vi "Get CDs NodeIDs by GUID.vi"(8 "error in (no error)":errorcluster, 10 "Custom Device GUID":string, 11 "Target ref in":refnum<k24>) -> (0 "error out":errorcluster, 2 "NodeIDs":u64[](array[numeric]), 3 "Target ref out":refnum<k24>)   [LabVIEW 2019, in "TLCD Test.lvclass"]
uses:
  TLCD Test.lvclass
  NationalInstruments.VeriStand.SystemDefinitionAPI
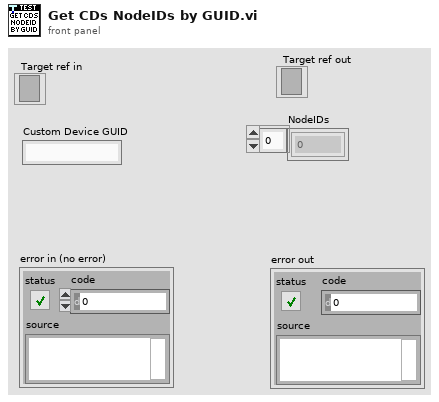
[diagram p1: front panel]
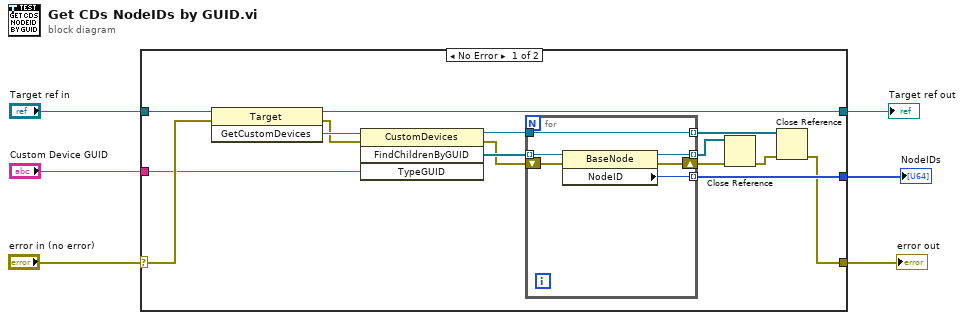
[diagram p0: block diagram]
diagram:
  n1 = case shown="No Error" "error in (no error)" {
    selector: "error in (no error)" -> [w20 w28]
    tunnel: "Target ref in" -> [w21 w29]
    tunnel: [w16 w29] -> w5
    tunnel: [w7 w28] -> w4
    tunnel: "Custom Device GUID" -> [w18 _]
    tunnel: [w13 _] -> w1
    frame No Error {
      n2 = invoke class="Target" method="GetCustomDevices"(reference=w21, error in=w20) -> (reference out=w16:refnum<k24>, error out=w17:errorcluster, "GetCustomDevices"=w19:refnum<k24>)  [unwired: 1 in]
      n3 = invoke class="CustomDevices" method="FindChildrenByGUID"(reference=w19, error in=w17, "TypeGUID"=w18) -> (reference out=w10:refnum<k24>, error out=w14:errorcluster, "FindChildrenByGUID"=w15:refnum<k24>[])  [unwired: 1 in, 1 out]
      n4 = for {
        tunnel: w15 -> [w27] mode=indexing
        tunnel: [w25] -> w13 mode=indexing
        shift-right: [w24] -> w12
        shift-left: w14 -> [w26]
        tunnel: [w23] -> w11 mode=indexing
        tunnel: w10 -> [w22]
        tunnel: [w22] -> w9 mode=indexing
        n5 = property class="BaseNode"(reference=w27, error in=w26) -> (reference out=w23:refnum<k24>, error out=w24:errorcluster, "NodeID"=w25:u64)
      }
      n6 = Close Reference(reference=w11, error in (no error)=w12) -> (error out=w8:errorcluster)
      n7 = Close Reference(reference=w9, error in (no error)=w8) -> (error out=w7:errorcluster)
    }
    frame Error {
    }
  }
  "Target ref out" <- w5
  "error out" <- w4
  "NodeIDs" <- w1
